vi "K2400_ApplyVOLTsafe_GUMS.vi"(1 "Voltage target [V]":dbl, 2 "VISA Resource Name":refnum<visa-resource-name>="GPIB0::11::INSTR") -> ()   [LabVIEW 2011]
uses:
  GlobalVar.vi
panel:
  out "Sweep":bool=TRUE
  out "V step [V]":dbl=0.001
  in  "Voltage temp [V]":dbl=0.06499999999999999
  out "Voltage init [V]":dbl=-0.001665
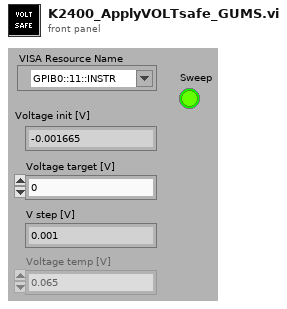
[diagram p1: front panel]
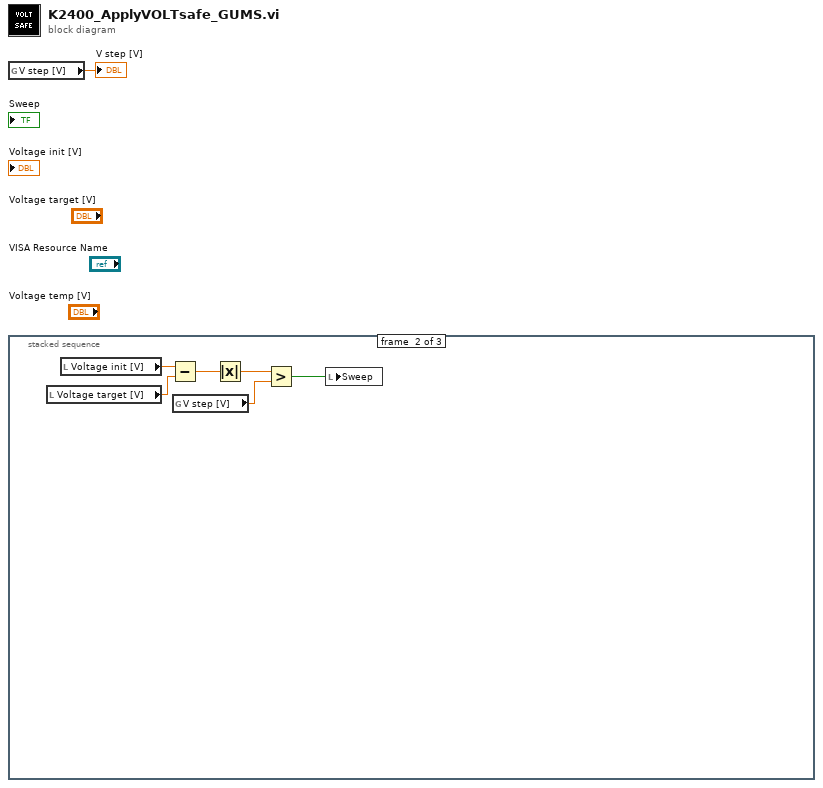
[diagram p0: block diagram]
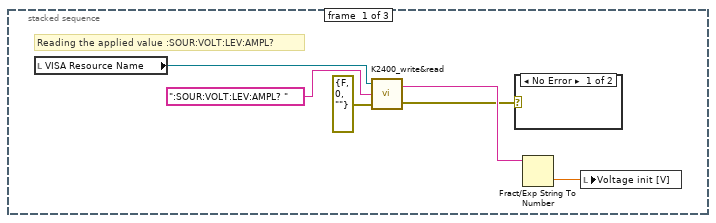
[diagram p2: hidden frame]
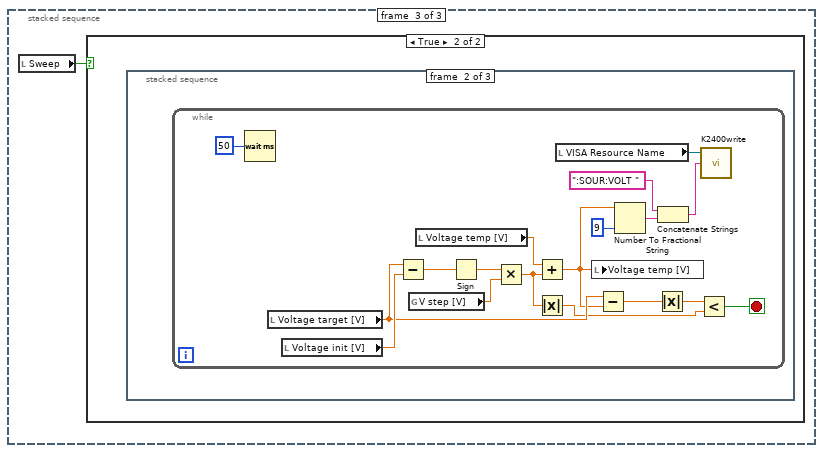
[diagram p4: hidden frame]
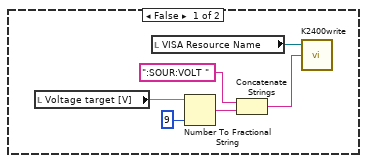
[diagram p5: hidden frame]
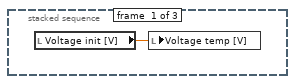
[diagram p6: hidden frame]
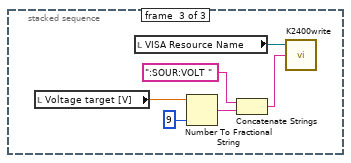
[diagram p7: hidden frame]
diagram:
  n1 = global read "GlobalVar.vi" "V step [V]"() -> (→"V step [V]":dbl)
  n2 = stacked-sequence {
    frame #0 {
      # "Reading the applied value :SOUR:VOLT:LEV:AMPL?"
      n3 = local read "VISA Resource Name"() -> (w5:refnum<visa-resource-name>)
      n4 = call "K2400_write&read.vi"("error in (no error)"=errorcluster {"status"=FALSE, "code"=0, "source"=""}, "Command"=":SOUR:VOLT:LEV:AMPL? ", "VISA Resource Name"=w5) -> ("error out"=w3:errorcluster, "Read"=w4:string)
      n5 = case shown="No Error" w3 {
        frame No Error {
        }
        frame Error {
        }
      }
      n6 = Fract/Exp String To Number(string=w4) -> (number=w7:dbl)  [unwired: 4 out]
      n7 = local write "Voltage init [V]"(w7) -> ()
    }
    frame #1 {
      n8 = local read "Voltage target [V]"() -> (w9:dbl)
      n9 = local read "Voltage init [V]"() -> (w10:dbl)
      n10 = Subtract(x=w10, y=w9) -> (x-y=w13:dbl)
      n11 = global read "GlobalVar.vi" "V step [V]"() -> (w8:dbl)
      n12 = Absolute Value(x=w13) -> (abs(x)=w12:dbl)
      n13 = Greater?(x=w12, y=w8) -> (0:w11:bool)
      n14 = local write "Sweep"(w11) -> ()
    }
    frame #2 {
      n15 = local read "Sweep"() -> (w14:bool)
      n16 = case shown="True" w14 {
        frame False {
          n17 = local read "Voltage target [V]"() -> (w17:dbl)
          n18 = local read "VISA Resource Name"() -> (w15:refnum<visa-resource-name>)
          n19 = Number To Fractional String(number=w17, precision (6)=9) -> (F-format string=w20:string)  [unwired: 2 out]
          n20 = Concatenate Strings(":SOUR:VOLT ", w20) -> (w16:string)
          n21 = call "K2400write.vi"("Command"=w16, "VISA Resource Name"=w15) -> ()  [unwired: 1 in, 2 out]
        }
        frame True {
          n22 = stacked-sequence {
            frame #0 {
              n23 = local read "Voltage init [V]"() -> (w21:dbl)
              n24 = local write "Voltage temp [V]"(w21) -> ()
            }
            frame #1 {
              n25 = while {
                stop <- w28 stop-if-true
                n26 = Wait (ms)(milliseconds to wait=50) -> ()  [unwired: 1 out]
                n27 = local read "Voltage target [V]"() -> (w32:dbl)
                n28 = local read "Voltage init [V]"() -> (w37:dbl)
                n29 = Subtract(x=w32, y=w37) -> (x-y=w39:dbl)
                n30 = global read "GlobalVar.vi" "V step [V]"() -> (w22:dbl)
                n31 = local read "Voltage temp [V]"() -> (w36:dbl)
                n32 = Sign(1:w39) -> (0:w38:dbl)
                n33 = Multiply(x=w38, y=w22) -> (x*y=w24:dbl)
                n34 = Add(x=w36, y=w24) -> (x+y=w31:dbl)
                n35 = Absolute Value(x=w24) -> (abs(x)=w23:dbl)
                n36 = local read "VISA Resource Name"() -> (w25:refnum<visa-resource-name>)
                n37 = local write "Voltage temp [V]"(w31) -> ()
                n38 = Subtract(x=w32, y=w31) -> (x-y=w30:dbl)
                n39 = Number To Fractional String(number=w31, precision (6)=9) -> (F-format string=w35:string)  [unwired: 2 out]
                n40 = Absolute Value(x=w30) -> (abs(x)=w29:dbl)
                n41 = Concatenate Strings(":SOUR:VOLT ", w35) -> (w26:string)
                n42 = Less?(x=w29, y=w23) -> (x < y?=w28:bool)
                n43 = call "K2400write.vi"("Command"=w26, "VISA Resource Name"=w25) -> ()  [unwired: 1 in, 2 out]
              }
            }
            frame #2 {
              n44 = local read "Voltage target [V]"() -> (w42:dbl)
              n45 = local read "VISA Resource Name"() -> (w40:refnum<visa-resource-name>)
              n46 = Number To Fractional String(number=w42, precision (6)=9) -> (F-format string=w45:string)  [unwired: 2 out]
              n47 = Concatenate Strings(":SOUR:VOLT ", w45) -> (w41:string)
              n48 = call "K2400write.vi"("Command"=w41, "VISA Resource Name"=w40) -> ()  [unwired: 1 in, 2 out]
            }
          }
        }
      }
    }
  }
